vi "Open.vi"(8 "error in (no error)":errorcluster, 11 "ENET In":refnum<class "ENET_BS120x.lvclass">) -> (0 "error out":errorcluster, 3 "ENET out":refnum<class "ENET_BS120x.lvclass">)   [LabVIEW 2021, in "BS120x Driver.lvlib" / "ENET_BS120x.lvclass"]
doc: "Open an Ethernet connection to the Battery Simulator 1200 at the specified IP address and ports.\n(c) 2019 Bloomy Controls, Inc. All rights reserved."
uses:
  ENET_BS120x.lvclass
  ENET_BS120x.lvclass/ENET_BS120x.ctl
  Async Heartbeat.vi
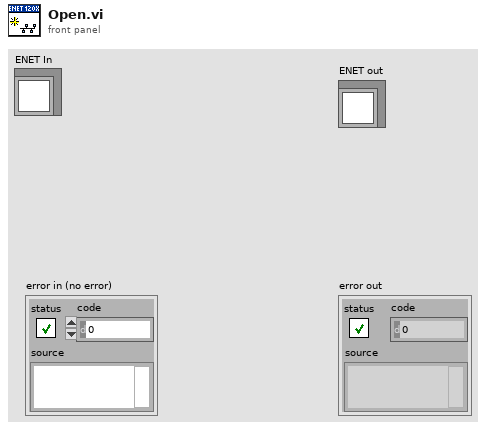
[diagram p1: front panel]
types:
  T1 = typedef "BS120x Driver.lvlib/BS120x.lvclass/Ethernet Settings.ctl" = cluster{"IP Address":string, "TCP (Command) Port":u16, "TCP (Command) Read Interval (ms)":u32, "UDP (Reporting) Port":u16, "UDP (Reporting) Write Interval (ms)":u32, "UDP Data Broadcast Enable":bool}
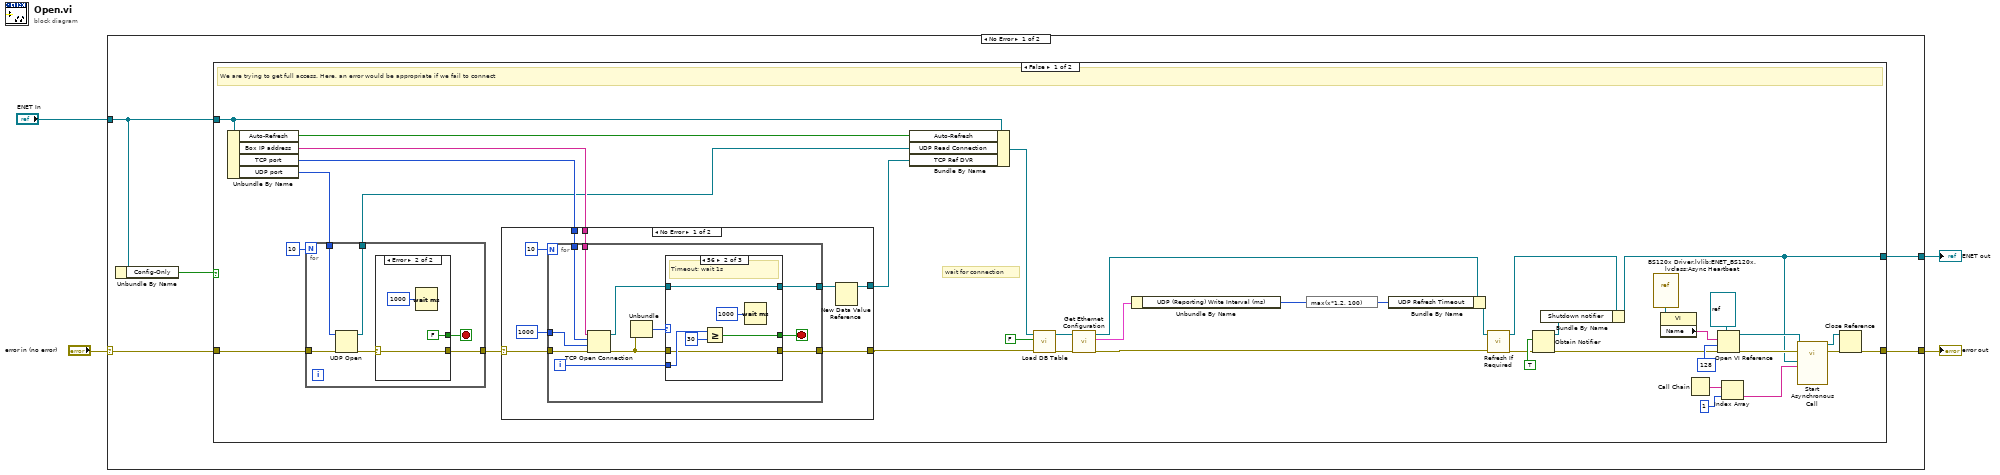
[diagram p0: block diagram]
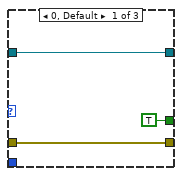
[diagram p2: hidden frame]
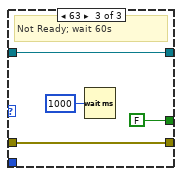
[diagram p3: hidden frame]
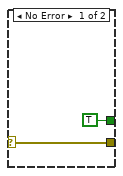
[diagram p5: hidden frame]
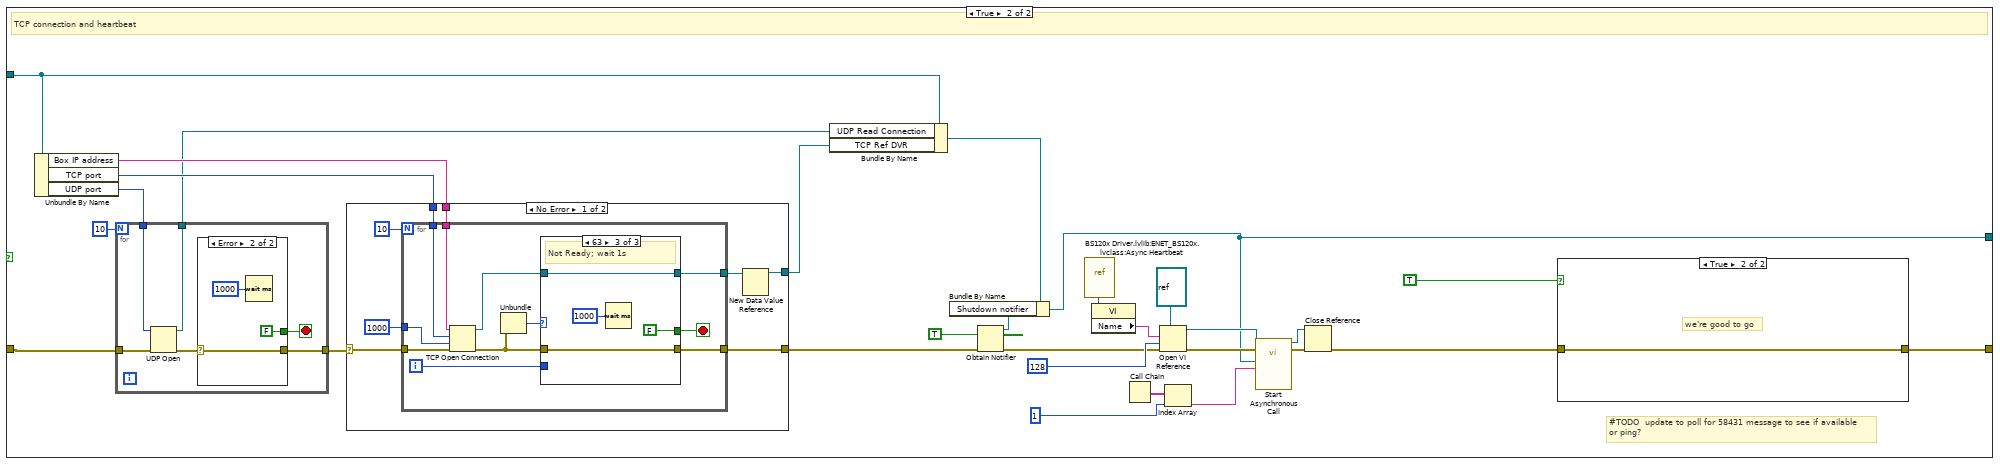
[diagram p6: hidden frame]
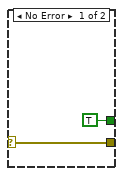
[diagram p7: hidden frame]
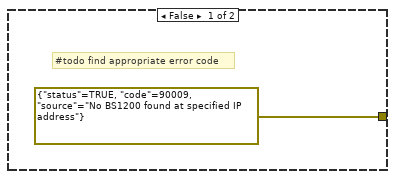
[diagram p8: hidden frame]
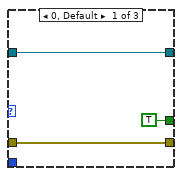
[diagram p9: hidden frame]
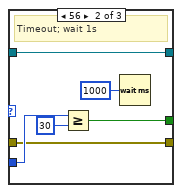
[diagram p10: hidden frame]
diagram:
  n1 = case shown="No Error" "error in (no error)" {
    selector: "error in (no error)" -> [w7 w169]
    tunnel: [w8 w169] -> w3
    tunnel: [w9 w168] -> w2
    tunnel: "ENET In" -> [w6 w168]
    frame No Error {
      n2 = Unbundle By Name(w6) -> ("Config-Only"=w5:bool)
      n3 = case shown="False" w5 {
        tunnel: [w19 w99] -> w9
        tunnel: [w23 w120] -> w8
        tunnel: w6 -> [w16 w116]
        tunnel: w7 -> [w37 w95]
        frame False {
          # "wait for connection"
          # "We are trying to get full access. Here, an error would be appropriate if we fail to connect"
          n4 = Unbundle By Name(w16) -> ("Auto-Refresh"=w10:bool, "Box IP address"=w47:string, "TCP port"=w46:u16, "UDP port"=w45:u16)
          n5 = for {
            N: 10 -> [_]
            tunnel: w45 -> [w86]
            tunnel: [w85] -> w13
            tunnel: w37 -> [w87]
            tunnel: [w83] -> w36
            stop <- w82 stop-if-true
            n6 = UDP Open(8:w87, 11:w86) -> (port=w85:refnum<k16>, 0:w84:errorcluster)  [unwired: 3 in, 1 out]
            n7 = case shown="Error" w84 {
              selector: w84 -> [w89 w91]
              tunnel: [w89 w91] -> w83
              tunnel: [TRUE FALSE] -> w82
              frame No Error {
              }
              frame Error {
                n8 = Wait (ms)(milliseconds to wait=u32 1000) -> ()  [unwired: 1 out]
              }
            }
          }
          n9 = case shown="No Error" w36 {
            selector: w36 -> [w52 w81]
            tunnel: w47 -> [w56 _]
            tunnel: w46 -> [w55 _]
            tunnel: [w51 w81] -> w11
            tunnel: [w49 _] -> w14
            frame No Error {
              n10 = for {
                N: 10 -> [_]
                tunnel: w56 -> [w66]
                tunnel: w55 -> [w65]
                tunnel: 1000 ("timeout ms (25000)") -> [w64]
                tunnel: w52 -> [w67]
                tunnel: [w60] -> w51
                tunnel: [w57] -> w50
                i -> [w63]
                stop <- w62 stop-if-true
                n11 = TCP Open Connection(address=w66, remote port or service name=w65, timeout ms (60000)=w64, error in (no error)=w67) -> (connection ID=w58:refnum<k5>, error out=w59:errorcluster)  [unwired: 1 in]
                n12 = Unbundle(w59) -> ("code"=w61:i32)  [unwired: 2 out]
                n13 = case shown="56" w61 {
                  tunnel: w63 -> [_ w75 _]
                  tunnel: [TRUE w73 FALSE] -> w62
                  tunnel: [w69 w72 w78] -> w60
                  tunnel: w59 -> [w69 w72 w78]
                  tunnel: w58 -> [w68 w71 w77]
                  tunnel: [w68 w71 w77] -> w57
                  frame 0, Default {
                  }
                  frame 56 {
                    # "Timeout; wait 1s"
                    n14 = Greater Or Equal?(x=w75, y=30 ("x")) -> (x >= y?=w73:bool)
                    n15 = Wait (ms)(milliseconds to wait=u32 1000) -> ()  [unwired: 1 out]
                  }
                  frame 63 {
                    # "Not Ready; wait 60s"
                    n16 = Wait (ms)(milliseconds to wait=u32 1000) -> ()  [unwired: 1 out]
                  }
                }
              }
              n17 = New Data Value Reference(data value=w50) -> (data value reference=w49:refnum<data-value>)  [unwired: 1 in, 1 out]
            }
            frame Error {
            }
          }
          n18 = Bundle By Name(cluster=w16, "Auto-Refresh"=w10, "UDP Read Connection"=w13, "TCP Ref DVR"=w14) -> (w15:refnum<class "ENET_BS120x.lvclass">)
          n19 = call-dynamic "Load DB Table.vi"("error in (no error)"=w11, "Calibration Mode"=FALSE, "ENET in"=w15) -> ("error out"=w43:errorcluster, "ENET out"=w44:refnum<class "ENET_BS120x.lvclass">)  [unwired: 7 in]
          n20 = call-dynamic "Get Ethernet Configuration.vi"("error in (no error)"=w43, "BS120x in"=w44) -> ("error out"=w12:errorcluster, "Ethernet Settings"=w17:T1, "BS120x out"=w42:refnum<class "ENET_BS120x.lvclass">)  [unwired: 6 in, 1 out]
          n21 = Unbundle By Name(w17) -> ("UDP (Reporting) Write Interval (ms)"=w40:u32)
          n22 = expression code="max(x*1.2, 100)"(w40) -> (w39:u32)
          n23 = Bundle By Name(cluster=w42, "UDP Refresh Timeout"=w39) -> (w41:refnum<class "ENET_BS120x.lvclass">)
          n24 = call "Refresh If Required.vi"("error in (no error)"=w12, "Ethernet in"=w41) -> ("error out"=w22:errorcluster, "Ethernet out"=w20:refnum<class "ENET_BS120x.lvclass">)  [unwired: 8 in]
          n25 = Obtain Notifier(notification data type=TRUE, error in (no error)=w22) -> (notifier out=w21:refnum<notifier>, error out=w18:errorcluster)  [unwired: 2 in, 1 out]
          n26 = Bundle By Name(cluster=w20, "Shutdown notifier"=w21) -> (w19:refnum<class "ENET_BS120x.lvclass">)
          n27 = vi-ref "BS120x Driver.lvlib:ENET_BS120x.lvclass:Async Heartbeat.vi"() -> (w33:refnum<vi>)
          n28 = property class="VI"(reference=w33) -> ("Name"=w34:string)  [unwired: 1 in, 2 out]
          n29 = Call Chain() -> (call chain=w30:string[])
          n30 = Open VI Reference(type specifier VI Refnum (for type only)=refnum<vi> refnum ("VI Refnum"), vi path=w34, options=128, error in (no error)=w18) -> (vi reference=w27:refnum<vi>, error out=w26:errorcluster)  [unwired: 2 in]
          n31 = Index Array(array=w30, index=1) -> (element=w28:string)
          n32 = call-by-ref "Start Asynchronous Call"(reference=w27, error in=w26, "Main VI"=w28, "Ethernet out"=w19) -> (reference out=w24:refnum<vi>, error out=w25:errorcluster)  [unwired: 10 in]
          n33 = Close Reference(reference=w24, error in (no error)=w25) -> (error out=w23:errorcluster)
        }
        frame True {
          # "#TODO  update to poll for 58431 message to see if available\nor ping?"
          # "TCP connection and heartbeat"
          n34 = Unbundle By Name(w116) -> ("Box IP address"=w118:string, "TCP port"=w117:u16, "UDP port"=w94:u16)
          n35 = for {
            N: 10 -> [_]
            tunnel: w94 -> [w126]
            tunnel: [w125] -> w93
            tunnel: w95 -> [w127]
            tunnel: [w123] -> w96
            stop <- w122 stop-if-true
            n36 = UDP Open(8:w127, 11:w126) -> (port=w125:refnum<k16>, 0:w124:errorcluster)  [unwired: 3 in, 1 out]
            n37 = case shown="Error" w124 {
              selector: w124 -> [w129 w131]
              tunnel: [w129 w131] -> w123
              tunnel: [TRUE FALSE] -> w122
              frame No Error {
              }
              frame Error {
                n38 = Wait (ms)(milliseconds to wait=u32 1000) -> ()  [unwired: 1 out]
              }
            }
          }
          n39 = case shown="No Error" w96 {
            selector: w96 -> [w138 w167]
            tunnel: w118 -> [w142 _]
            tunnel: w117 -> [w141 _]
            tunnel: [w137 w167] -> w101
            tunnel: [w135 _] -> w119
            frame No Error {
              n40 = for {
                N: 10 -> [_]
                tunnel: w142 -> [w152]
                tunnel: w141 -> [w151]
                tunnel: 1000 ("timeout ms (25000)") -> [w150]
                tunnel: w138 -> [w153]
                tunnel: [w146] -> w137
                tunnel: [w143] -> w136
                i -> [w149]
                stop <- w148 stop-if-true
                n41 = TCP Open Connection(address=w152, remote port or service name=w151, timeout ms (60000)=w150, error in (no error)=w153) -> (connection ID=w144:refnum<k5>, error out=w145:errorcluster)  [unwired: 1 in]
                n42 = Unbundle(w145) -> ("code"=w147:i32)  [unwired: 2 out]
                n43 = case shown="63" w147 {
                  tunnel: w149 -> [_ w161 _]
                  tunnel: [TRUE w159 FALSE] -> w148
                  tunnel: [w155 w158 w164] -> w146
                  tunnel: w145 -> [w155 w158 w164]
                  tunnel: w144 -> [w154 w157 w163]
                  tunnel: [w154 w157 w163] -> w143
                  frame 0, Default {
                  }
                  frame 56 {
                    # "Timeout; wait 1s"
                    n44 = Greater Or Equal?(x=w161, y=30 ("x")) -> (x >= y?=w159:bool)
                    n45 = Wait (ms)(milliseconds to wait=u32 1000) -> ()  [unwired: 1 out]
                  }
                  frame 63 {
                    # "Not Ready; wait 1s"
                    n46 = Wait (ms)(milliseconds to wait=u32 1000) -> ()  [unwired: 1 out]
                  }
                }
              }
              n47 = New Data Value Reference(data value=w136) -> (data value reference=w135:refnum<data-value>)  [unwired: 1 in, 1 out]
            }
            frame Error {
            }
          }
          n48 = Bundle By Name(cluster=w116, "UDP Read Connection"=w93, "TCP Ref DVR"=w119) -> (w100:refnum<class "ENET_BS120x.lvclass">)
          n49 = Obtain Notifier(notification data type=TRUE, error in (no error)=w101) -> (notifier out=w103:refnum<notifier>, error out=w102:errorcluster)  [unwired: 2 in, 1 out]
          n50 = Bundle By Name(cluster=w100, "Shutdown notifier"=w103) -> (w99:refnum<class "ENET_BS120x.lvclass">)
          n51 = vi-ref "BS120x Driver.lvlib:ENET_BS120x.lvclass:Async Heartbeat.vi"() -> (w113:refnum<vi>)
          n52 = property class="VI"(reference=w113) -> ("Name"=w114:string)  [unwired: 1 in, 2 out]
          n53 = Call Chain() -> (call chain=w110:string[])
          n54 = Open VI Reference(type specifier VI Refnum (for type only)=refnum<vi> refnum ("VI Refnum"), vi path=w114, options=128, error in (no error)=w102) -> (vi reference=w107:refnum<vi>, error out=w106:errorcluster)  [unwired: 2 in]
          n55 = Index Array(array=w110, index=1) -> (element=w108:string)
          n56 = call-by-ref "Start Asynchronous Call"(reference=w107, error in=w106, "Main VI"=w108, "Ethernet out"=w99) -> (reference out=w104:refnum<vi>, error out=w105:errorcluster)  [unwired: 10 in]
          n57 = Close Reference(reference=w104, error in (no error)=w105) -> (error out=w98:errorcluster)
          n58 = case shown="True" TRUE {
            tunnel: w98 -> [_ w134]
            tunnel: [errorcluster {"status"=TRUE, "code"=90009, "source"="No BS1200 found at specified IP address"} ("error constant") w134] -> w120
            frame False {
              # "#todo find appropriate error code"
            }
            frame True {
              # "we're good to go"
            }
          }
        }
      }
    }
    frame Error {
    }
  }
  "error out" <- w3
  "ENET out" <- w2
